vi "CreateTelegramSubVI.vi"(2 "seconds":dbl min=0.0 max=59.0 step=1.0 format="%02d", 3 "minutes":dbl min=0.0 max=59.0 step=1.0 format="%02d", 4 "hours":dbl min=0.0 max=24.0 step=1.0 format="%02d", 5 "temperature":dbl min=0.0 max=400.0 step=1.0 format="%03d") -> (0 "tempTelegram":string)   [LabVIEW 2012]
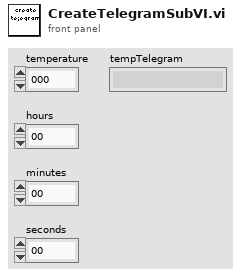
[diagram p1: front panel]
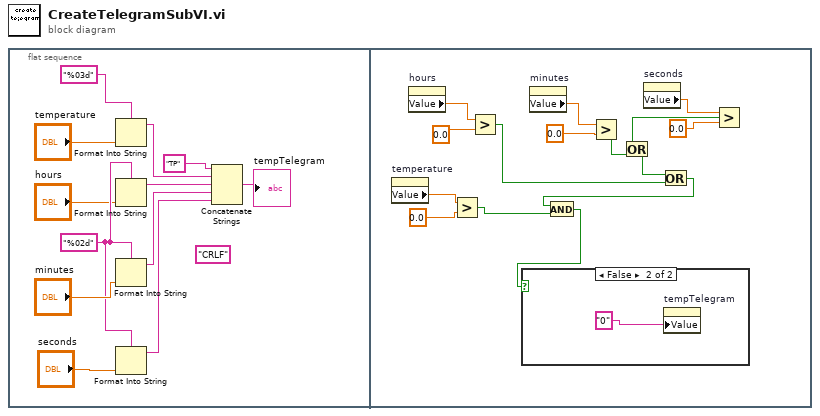
[diagram p0: block diagram]
diagram:
  n1 = flat-sequence {
    frame #0 {
      w8 = "%02d" ("format string")
      (unwired) "CRLF"
      n2 = Format Into String(format string="%03d", "temperature") -> (resulting string=w6:string)  [unwired: 2 in, 1 out]
      n3 = Format Into String(format string=w8, "hours") -> (resulting string=w3:string)  [unwired: 2 in, 1 out]
      n4 = Format Into String(format string=w8, "minutes") -> (resulting string=w11:string)  [unwired: 2 in, 1 out]
      n5 = Format Into String(format string=w8, "seconds") -> (resulting string=w12:string)  [unwired: 2 in, 1 out]
      n6 = Concatenate Strings("TP", w6, w3, w11, w12) -> (→"tempTelegram":string)
    }
    frame #1 {
      n7 = property on="temperature" class="DigNum (strict)"() -> ("Value"=w25:dbl)  [unwired: 2 in, 2 out]
      n8 = property on="hours" class="DigNum (strict)"() -> ("Value"=w27:dbl)  [unwired: 2 in, 2 out]
      n9 = Greater?(x=w25, y=0.0) -> (0:w19:bool)
      n10 = Greater?(x=w27, y=0.0) -> (0:w13:bool)
      n11 = property on="minutes" class="DigNum (strict)"() -> ("Value"=w21:dbl)  [unwired: 2 in, 2 out]
      n12 = Greater?(x=w21, y=0.0) -> (0:w16:bool)
      n13 = property on="seconds" class="DigNum (strict)"() -> ("Value"=w23:dbl)  [unwired: 2 in, 2 out]
      n14 = Greater?(x=w23, y=0.0) -> (0:w15:bool)
      n15 = Or(x=w15, y=w16) -> (x .or. y?=w14:bool)
      n16 = Or(x=w14, y=w13) -> (x .or. y?=w18:bool)
      n17 = And(x=w18, y=w19) -> (x .and. y?=w17:bool)
      n18 = case shown="False" w17 {
        frame True {
        }
        frame False {
          n19 = property on="tempTelegram" class="Str"("Value"="0" ("tempTelegram")) -> ()  [unwired: 2 in, 2 out]
        }
      }
    }
  }
